vi "StackLocation.vi"(11 "Mode":T1(ring)=enum."Retrieve Stack Location") -> (2 "Current\nWindDirection":dbl, 3 "StackPosition (at 0deg)":sgl[](array[numeric]))   [LabVIEW 2018]
uses:
  ADAM Client/Sub VIs/ADAM Controls/Update_scan_value.ctl
  Trav_mode.ctl
  Controls/User_Specific_mode.ctl
  Controls/Tunnel_Coordinates.ctl
  Globals/Preference_global.vi
  Globals/Trav_pos_global.vi
panel:
  in  "Extra Command String":string
  out "MeasuredStackPosition":sgl[](array[numeric]) format="%.2f"
  # "• First, check the probe is correctly zeroed at TT centre.\n• Next, position the probe directly over the stack under study, with the turntable at any angle you like.\n• Then select \"Record Stack Location\" mode, and run this VI."
  # "@"
  # "="
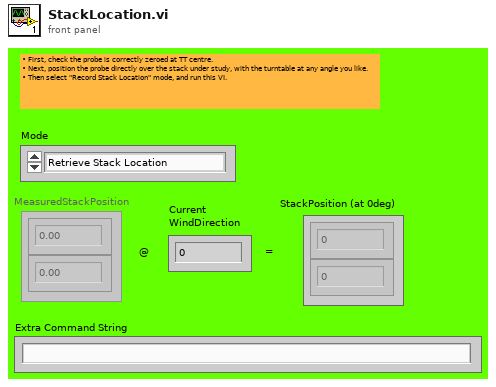
[diagram p1: front panel]
types:
  T1 = enum16{"Record Stack Location", "Retrieve Stack Location"}
  T2 = typedef "Tunnel_Coordinates.ctl" = enum16{"Work in Tunnel Coordinates", "Work in Model Coordinates"}
  T3 = enum8{"Enabled", "Disabled", "Disabled and Grayed Out"}
  T4 = typedef "User_Specific_mode.ctl" = enum16{"Check VI only", "Run VI"}
  T5 = typedef "Trav_mode.ctl" = enum16{"Move traverse", "Read traverse position", "Teach Position"}
  T6 = typedef "Update_scan_value.ctl" = cluster{"Channel Name":string, "New Value":dbl}
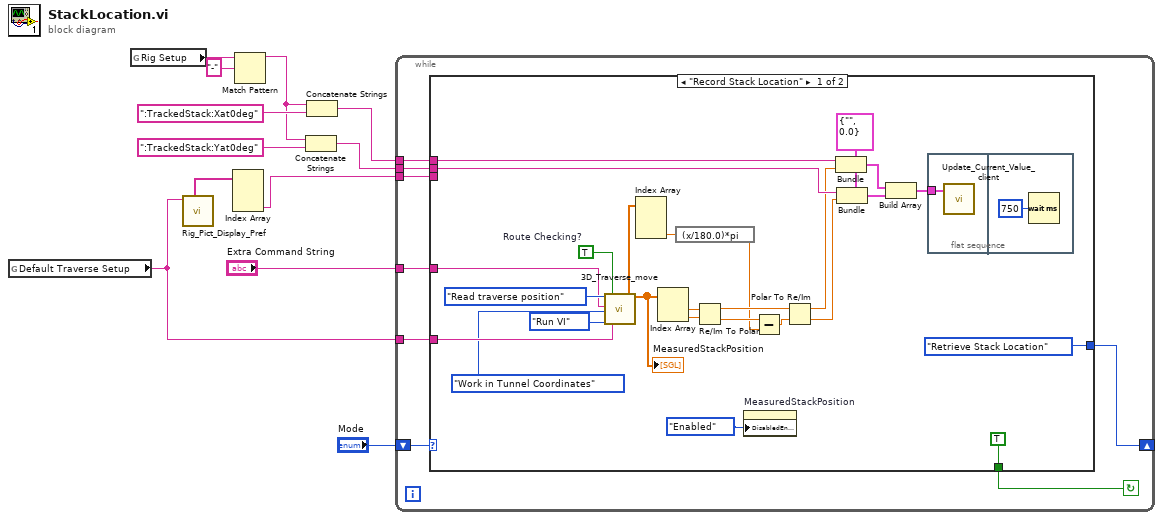
[diagram p0: block diagram]
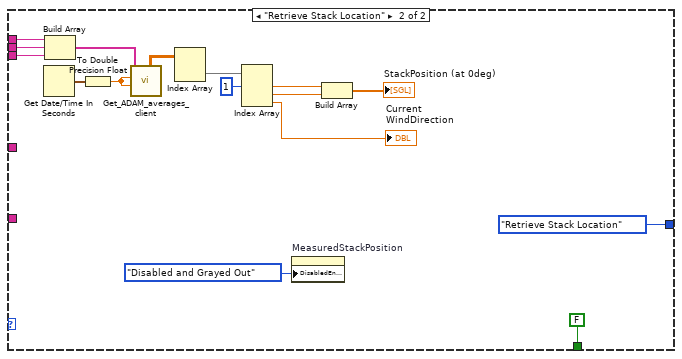
[diagram p2: hidden frame]
diagram:
  n1 = global read "Trav_pos_global.vi" "Default Traverse Setup"() -> (w4:string)
  n2 = global read "Preference_global.vi" "Rig Setup"() -> (w9:string)
  n3 = call "Rig_Pict_Display_Pref.vi"("Traverse Name"=w4) -> ("Roll Pitch Yaw ADAM Channels"=w3:string[])  [unwired: 3 in, 4 out]
  n4 = Index Array(array=w3) -> (element #3=w2:string)  [unwired: 3 in, 2 out]
  n5 = Match Pattern(string=w9, regular expression="-") -> (before substring=w8:string)  [unwired: 4 out]
  n6 = Concatenate Strings(w8, ":TrackedStack:Yat0deg") -> (w6:string)
  n7 = Concatenate Strings(w8, ":TrackedStack:Xat0deg") -> (w5:string)
  n8 = while {
    shift-right: [w18] -> _
    shift-left: "Mode" -> [w20]
    tunnel: w2 -> [w17]
    tunnel: w6 -> [w16]
    tunnel: w5 -> [w15]
    tunnel: w4 -> [w14]
    tunnel: "Extra Command String" -> [w13]
    stop <- w19 continue-if-true
    n9 = case shown="\"Record Stack Location\"" w20 {
      tunnel: [TRUE FALSE] -> w19
      tunnel: [T1."Retrieve Stack Location" ("Mode") T1."Retrieve Stack Location" ("Mode")] -> w18
      tunnel: w17 -> [_ w52]
      tunnel: w16 -> [w42 w51]
      tunnel: w15 -> [w43 w50]
      tunnel: w14 -> [w25 _]
      tunnel: w13 -> [w23 _]
      frame "Record Stack Location" {
        w21 = TRUE  # Route Checking?
        w44 = T6 {"Channel Name"="", "New Value"=0.0} ("Update Scan Value Cluster")
        n10 = call "3D_Traverse_move.vi"("Mode"=Trav_mode."Read traverse position", "Extra command String"=w23, "Work in Tunnel Coordinates"=Tunnel_Coordinates."Work in Tunnel Coordinates", "Simulate/Run"=User_Specific_mode."Run VI", "Route Checking?"=w21, "Traverse name"=w25) -> ("Model:    Roll        Pitch         Yaw  (deg)"=w27:sgl[], "Trav Position achieved"=w36:sgl[])  [unwired: 10 in, 2 out]
        "MeasuredStackPosition" <- w36
        n11 = Index Array(array=w27) -> (element #3=w26:sgl)  [unwired: 3 in, 2 out]
        n12 = Index Array(array=w36) -> (element #1=w31:sgl, element #2=w30:sgl)  [unwired: 2 in]
        n13 = expression code="(x/180.0)*pi" ("degrees to radians")(w26) -> (w32:sgl)
        n14 = Re/Im To Polar(2:w30, 3:w31) -> (0:w34:sgl, 1:w35:sgl)
        n15 = property on="MeasuredStackPosition" class="Arr (strict)"("DisabledEnum"=T3."Enabled" ("Disabled")) -> ()  [unwired: 2 in, 2 out]
        n16 = Subtract(x=w34, y=w32) -> (x-y=w33:sgl)
        n17 = Polar To Re/Im(2:w33, 3:w35) -> (0:w28:sgl, 1:w29:sgl)
        n18 = Bundle(cluster=w44, "Channel Name"=w43, "New Value"=w29) -> (w40:T6)
        n19 = Bundle(cluster=w44, "Channel Name"=w42, "New Value"=w28) -> (w41:T6)
        n20 = Build Array(w40, w41) -> (w39:T6[])
        n21 = flat-sequence {
          tunnel: w39 -> [w47]
          frame #0 {
            n22 = call "Update_Current_Value_client.vi"("Update array in"=w47) -> ()  [unwired: 1 in]
          }
          frame #1 {
            n23 = Wait (ms)(milliseconds to wait=u32 750) -> ()  [unwired: 1 out]
          }
        }
      }
      frame "Retrieve Stack Location" {
        n24 = Get Date/Time In Seconds() -> (seconds since 1Jan1904=w62:timestamp)
        n25 = Build Array(w50, w51, w52) -> (w53:string[])
        n26 = To Double Precision Float(number=w62) -> (double precision float=w61:dbl)
        n27 = call "Get_ADAM_averages_client.vi"("End time"=w61, "Start time"=w61, "ADAM Ch Names"=w53) -> ("DBL values"=w60:dbl[][])  [unwired: 2 in, 6 out]
        n28 = Index Array(array=w60) -> (element=w59:dbl[])  [unwired: 2 in]
        n29 = Index Array(array=w59, index #1=1 ("index")) -> (element #1=w57:dbl, element #2=w56:dbl, element #3=→"Current\nWindDirection":dbl)  [unwired: 2 in]
        n30 = property on="MeasuredStackPosition" class="Arr (strict)"("DisabledEnum"=T3."Disabled and Grayed Out" ("Disabled")) -> ()  [unwired: 2 in, 2 out]
        n31 = Build Array(w57, w56) -> (→"StackPosition (at 0deg)":dbl[])
      }
    }
  }
